vi "Clamp Wrapper.vi"(0 "In or Out":bool) -> ()   [LabVIEW 2014]
uses:
  Precreated VIs/Robot Global Data.vi
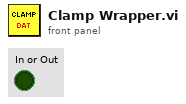
[diagram p1: front panel]
types:
  T1 = cluster{"Pickup Mechanism":cluster{"Lift":cluster{"Top":bool, "3":bool, "2":bool, "1":bool, "Bottom":bool}, "Clamp":cluster{"Widest":bool, "Narrowest":bool, "Left Arm":bool, "Right Arm":bool}}, "Ultrasonic":dbl, "Clamper Wide Tote":bool, "Tote in?":bool, "Lift Encoder":cluster{"Distance":dbl, "Rate":dbl, "Direction":bool, "Stopped":bool}, "Drive Encoders":cluster{"Distance":dbl, "Rate":dbl, "Direction":bool, "Stopped":bool}[]}
  T2 = cluster{"Widest":bool, "Narrowest":bool, "Left Arm":bool, "Right Arm":bool}
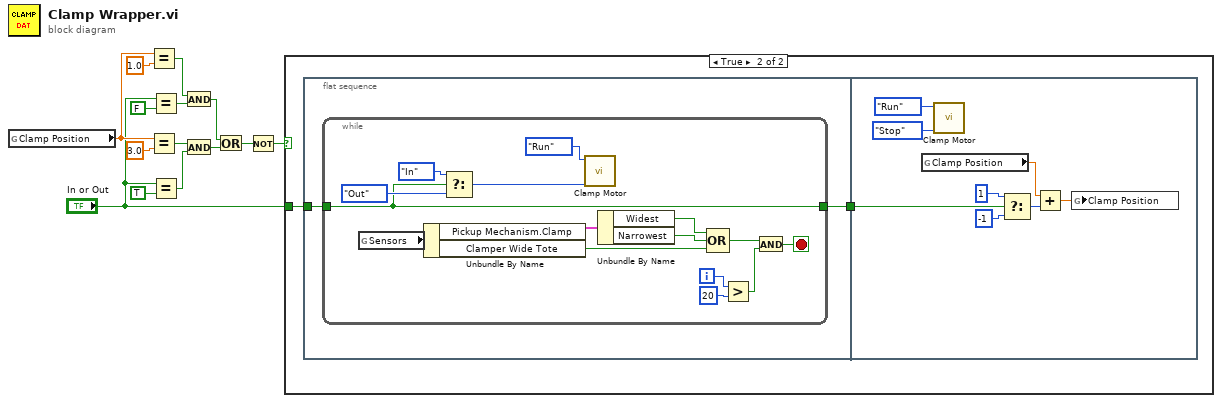
[diagram p0: block diagram]
diagram:
  n1 = global read "Robot Global Data.vi" "Clamp Position"() -> (w11:dbl)
  n2 = Equal?(x=w11, y=1.0) -> (x = y?=w9:bool)
  n3 = Equal?(x=w11, y=3.0) -> (x = y?=w6:bool)
  n4 = Equal?(x="In or Out", y=FALSE) -> (x = y?=w12:bool)
  n5 = Equal?(x="In or Out", y=TRUE) -> (x = y?=w7:bool)
  n6 = And(x=w9, y=w12) -> (x .and. y?=w5:bool)
  n7 = And(x=w6, y=w7) -> (x .and. y?=w4:bool)
  n8 = Or(x=w5, y=w4) -> (x .or. y?=w2:bool)
  n9 = Not(x=w2) -> (.not. x?=w3:bool)
  n10 = case shown="True" w3 {
    tunnel: "In or Out" -> [_ w16]
    frame False {
    }
    frame True {
      n11 = flat-sequence {
        tunnel: w16 -> [w18]
        tunnel: [w17] -> w15
        tunnel: w15 -> [w34]
        frame #0 {
          n12 = while {
            tunnel: w18 -> [w19]
            tunnel: [w19] -> w17
            i -> [w33]
            stop <- w24 stop-if-true
            n13 = global read "Robot Global Data.vi" "Sensors"() -> (w21:T1)
            n14 = Unbundle By Name(w21) -> ("Pickup Mechanism.Clamp"=w27:T2, "Clamper Wide Tote"=w20:bool)
            n15 = Select(t=enum16{"Stop", "In", "Out"}."In" ("Direction"), s=w19, f=enum16{"Stop", "In", "Out"}."Out" ("Direction")) -> (s? t:f=w30:enum16{"Stop", "In", "Out"})
            n16 = call "Clamp Motor.vi"("Direction"=w30, "Mode"=enum8{"Start", "Run", "Finish"}."Run") -> ()  [unwired: 2 in]
            n17 = Unbundle By Name(w27) -> ("Widest"=w28:bool, "Narrowest"=w29:bool)
            n18 = Compound Arithmetic op=OR(w28, w29, w20) -> (w26:bool)
            n19 = Greater?(x=w33, y=20) -> (0:w25:bool)
            n20 = And(x=w26, y=w25) -> (x .and. y?=w24:bool)
          }
        }
        frame #1 {
          n21 = global read "Robot Global Data.vi" "Clamp Position"() -> (w41:dbl)
          n22 = call "Clamp Motor.vi"("Direction"=enum16{"Stop", "In", "Out"}."Stop", "Mode"=enum8{"Start", "Run", "Finish"}."Run") -> ()  [unwired: 2 in]
          n23 = Select(t=1, s=w34, f=-1) -> (s? t:f=w37:i32)
          n24 = Add(x=w41, y=w37) -> (x+y=w40:dbl)
          n25 = global write "Robot Global Data.vi" "Clamp Position"(w40) -> ()
        }
      }
    }
  }
